vi "Initialize.vi"(7 "writer buffer size":i32=4096, 8 "error in (no error)":errorcluster, 9 "connection timeout":i32=-1, 10 "reader url":string, 11 "writer name":string) -> (0 "error out":errorcluster, 1 "Initialized?":bool, 3 "NetworkStreamWriter out":refnum<class "NetworkStreamWriter.lvclass">)   [LabVIEW 2011, in "NetworkStreamWriter.lvclass"]
doc: "This VI returns an instance of the NetworkStreamWriter class. A NetworkStreamWriter attempts to open a network stream with a reader endpoint. As with network streams, the writer url on the reader or the reader url on the writer must be given before the connection can be made. Note that until a connection is made, this VI will not return. It will, however, stop on a commanded e-stop from the top-level VI. This VI also launches a writer daemon which constantly sends information added to the internal queue by the Write method across the network stream."
uses:
  NetworkStreamWriter.lvclass
  Shared/message.ctl
  Shared/messageQueue.ctl
  NetworkStreamWriter.lvclass/NetworkStreamWriter.ctl
  WriterDaemon.vi
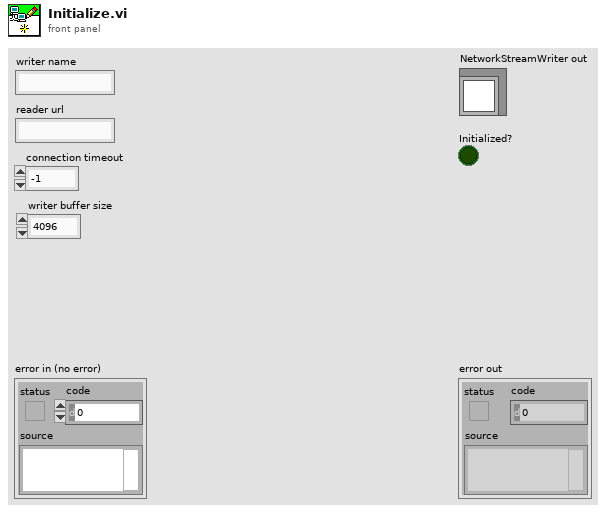
[diagram p1: front panel]
types:
  T1 = typedef "messageQueue.ctl" = refnum<queue>
  T2 = typedef "message.ctl" = cluster{"Data":variant, "Time since start (s)":dbl}
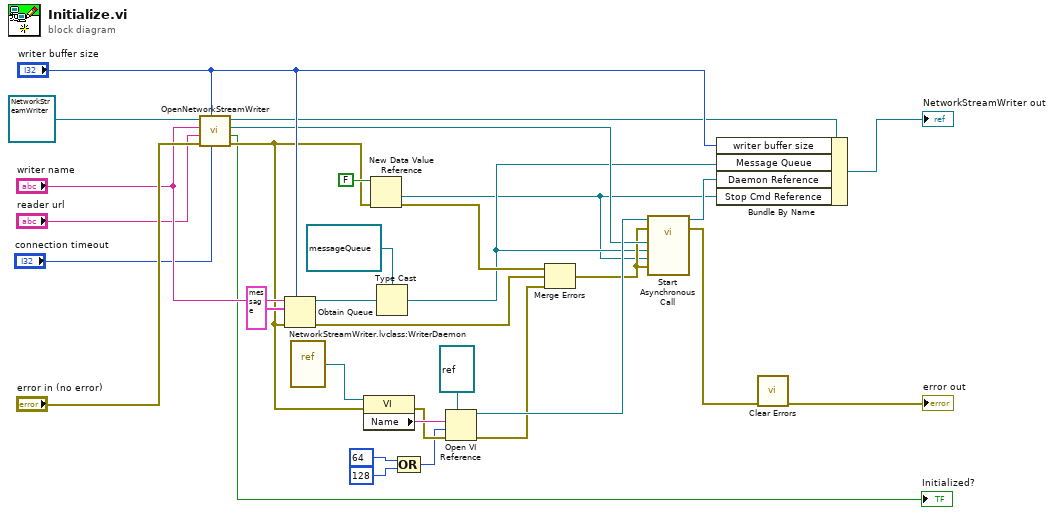
[diagram p0: block diagram]
diagram:
  n1 = call "OpenNetworkStreamWriter.vi"("connection timeout"="connection timeout", "writer buffer size"="writer buffer size", "error in (no error)"="error in (no error)", "reader url"="reader url", "writer name"="writer name", "NetworkStreamWriter in"=refnum<class "NetworkStreamWriter.lvclass"> refnum) -> ("error out"=w4:errorcluster, "Initialized?"=→"Initialized?":bool, "Writer Endpoint"=w17:refnum<k21>, "NetworkStreamWriter out"=w5:refnum<class "NetworkStreamWriter.lvclass">)  [unwired: 2 in]
  n2 = Obtain Queue(max queue size (-1, unlimited)="writer buffer size", name (unnamed)="writer name", element data type=T2 {"Data"=variant, "Time since start (s)"=0.0}, error in (no error)=w4) -> (queue out=w9:refnum<queue>, error out=w18:errorcluster)  [unwired: 1 in, 1 out]
  n3 = vi-ref "NetworkStreamWriter.lvclass:WriterDaemon.vi"() -> (w24:refnum<vi>)
  n4 = property class="VI"(reference=w24, error in=w4) -> (error out=w20:errorcluster, "Name"=w23:string)  [unwired: 1 out]
  n5 = New Data Value Reference(data value=FALSE, error in=w4) -> (data value reference=w6:refnum<data-value>, error out=w10:errorcluster)
  n6 = Type Cast(type=T1 refnum ("Variant Queue"), x=w9) -> (*(type *) &x=w7:T1)
  n7 = Compound Arithmetic op=OR(64 ("options"), 128 ("options")) -> (w12:i32)
  n8 = Open VI Reference(type specifier VI Refnum (for type only)=refnum<vi> refnum, vi path=w23, options=w12, error in (no error)=w20) -> (vi reference=w22:refnum<vi>, error out=w19:errorcluster)  [unwired: 2 in]
  n9 = Merge Errors(w10, w18, w19) -> (w16:errorcluster)
  n10 = call-by-ref "Start Asynchronous Call"(reference=w22, error in=w16, 8:"error in (no error)"=w16, "Stop Cmd Reference"=w6, "Message Queue"=w7, "Writer Endpoint"=w17) -> (reference out=w15:refnum<vi>, error out=w1:errorcluster)  [unwired: 8 in]
  n11 = Bundle By Name(cluster=w5, "writer buffer size"="writer buffer size", "Message Queue"=w7, "Daemon Reference"=w15, "Stop Cmd Reference"=w6) -> (→"NetworkStreamWriter out":refnum<class "NetworkStreamWriter.lvclass">)
  n12 = call <vilib>:"Clear Errors.vi"("error in (no error)"=w1) -> ("error out"=→"error out":errorcluster)  [unwired: 6 in]
